vi "Teleop.vi"(10 "Match Info":T3={"Autonomous Elapsed Seconds"=0.0, "TeleOp Elapsed Seconds"=0.0, "Disabled Elapsed Seconds"=0.0, "Visited Autonomous"=FALSE, "Visited TeleOp"=FALSE, "Visited Disabled"=FALSE, "Autonomous Settings"={"Autonomous Style"=enum."Independent", "VI Refnum"=refnum}}, 11 "Call Context":T4) -> ()   [LabVIEW 2017]
doc: "This VI is called for each TeleOp packet received from the DS where the robot is not disabled. It is often used to read from the joysticks and update I/O or to update setpoints for timed control loops. It should complete and return within 20 milliseconds or it may miss DS packets."
uses:
  <vilib>/Rock Robotics/WPI/DriverStation/WPI_DriverStationDerivedRobotMode.ctl
  <vilib>/Rock Robotics/WPI/DriverStation/WPI_DriverStationMatch Info.ctl
  <vilib>/Rock Robotics/WPI/ThirdParty/Phoenix-LabVIEW/Motor Controller/Controls/CTRE_Phoenix_MotorControl_ControlMode.ctl
  <vilib>/Rock Robotics/WPI/Utilities/WPI_GetSetVariantRefNum.vi
  <vilib>/Rock Robotics/WPI/ThirdParty/Phoenix-LabVIEW/Motor Controller/Get/CTRE_Phoenix_MotorController_GetSelectedSensorData.vi
panel:
  in  "newPosition":i32
  out "Velocity":T1(graph)
  out "Position":T2(graph)
  in  "windowSize":i32=1
  in  "Period":u16(ring)=100 items=["Period_1Ms"=1, "Period_2Ms"=2, "Period_5Ms"=5, "Period_10Ms"=10, "Period_20Ms"=20, "Period_25Ms"=25, "Period_50Ms"=50, "Period_100Ms"=100]
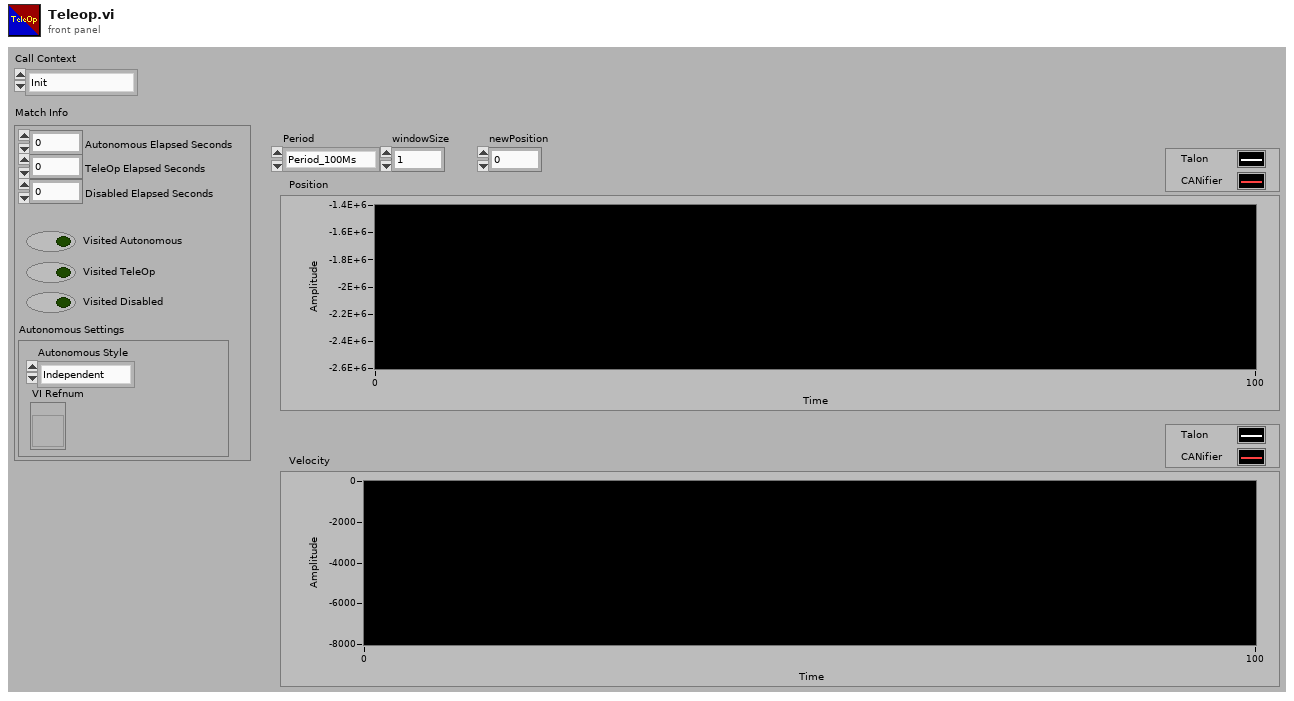
[diagram p1: front panel]
types:
  T1 = cluster{"Velocity (Raw Sensor Units per 100 ms)":i32, "vel":i32}
  T2 = cluster{"Position (Raw Sensor Units)":i32, "pos":i32}
  T3 = typedef "WPI_DriverStationMatch Info.ctl" = cluster{"Autonomous Elapsed Seconds":dbl, "TeleOp Elapsed Seconds":dbl, "Disabled Elapsed Seconds":dbl, "Visited Autonomous":bool, "Visited TeleOp":bool, "Visited Disabled":bool, "Autonomous Settings":cluster{"Autonomous Style":enum16{"Iterative", "Independent"}, "VI Refnum":refnum<vi>}}
  T4 = typedef "WPI_DriverStationDerivedRobotMode.ctl" = enum16{"Init", "Execute", "Stop"}
  T5 = typedef "CTRE_Phoenix_MotorControl_ControlMode.ctl" = u16
  T6 = typedef "WPI_JoystickDevRef.ctl" = cluster{"Device":T7}
  T7 = typedef "WPI_JoystickDeviceEnum.ctl" = enum16{"USB 0", "USB 1", "USB 2", "USB 3", "USB 4", "USB 5"}
  T8 = typedef "CTRE_CANifier_DeviceRef.ctl" = cluster{"DeviceStatus":errorcluster, "Device Number":u8, "Handle":u64, "UsageFrame":u32, "Library Path":path}
  T9 = typedef "WPI_MotorControlDeviceRef.ctl" = cluster{"DeviceStatus":errorcluster, "Type":T10, "PWM":cluster{"PWM Channel":T11, "DeadBand":T12}, "CAN":cluster{"Device Number":u8, "SetOutput VI Ref":variant, "GetOutput VI Ref":variant, "Enable VI Ref":variant, "Disable VI Ref":variant, "Data":variant}, "Invert":bool, "DIO PWM":cluster{"PWM \"Enable\" Channel":T11, "DIOChannel":T13, "PWM Rate":dbl}}
  T10 = typedef "WPI_MotorControlType.ctl" = enum16{"PWM", "CAN", "DIO PWM"}
  T11 = typedef "FPGA_DIOPWMChannel.ctl" = enum8{"PWM 0", "PWM 1", "PWM 2", "PWM 3", "PWM 4", "PWM 5", "PWM 6", "PWM 7", "PWM 8", "PWM 9", "PWM MXP 0", "PWM MXP 1", "PWM MXP 2", "PWM MXP 3", "PWM MXP 4", "PWM MXP 5", "PWM MXP 6", "PWM MXP 7", "PWM MXP 8", "PWM MXP 9", "Invalid"}
  T12 = typedef "WPI_PWMDeadband.ctl" = cluster{"Name":string, "maxPositivePwm":i32, "minPositivePwm":i32, "centerPwm":i32, "maxNegativePwm":i32, "minNegativePwm":i32, "angularRange":u16}
  T13 = typedef "FPGA_DIOChannel.ctl" = enum8{"DIO 0", "DIO 1", "DIO 2", "DIO 3", "DIO 4", "DIO 5", "DIO 6", "DIO 7", "DIO 8", "DIO 9", "DIO MXP 0", "DIO MXP 1", "DIO MXP 2", "DIO MXP 3", "DIO MXP 4", "DIO MXP 5", "DIO MXP 6", "DIO MXP 7", "DIO MXP 8", "DIO MXP 9", "DIO MXP 10", "DIO MXP 11", "DIO MXP 12", "DIO MXP 13", "DIO MXP 14", "DIO MXP 15", "SPI Port CS1", "SPI Port CS2", "SPI Port CS3", "SPI Port MISO", "SPI Port MOSI", "Invalid"}
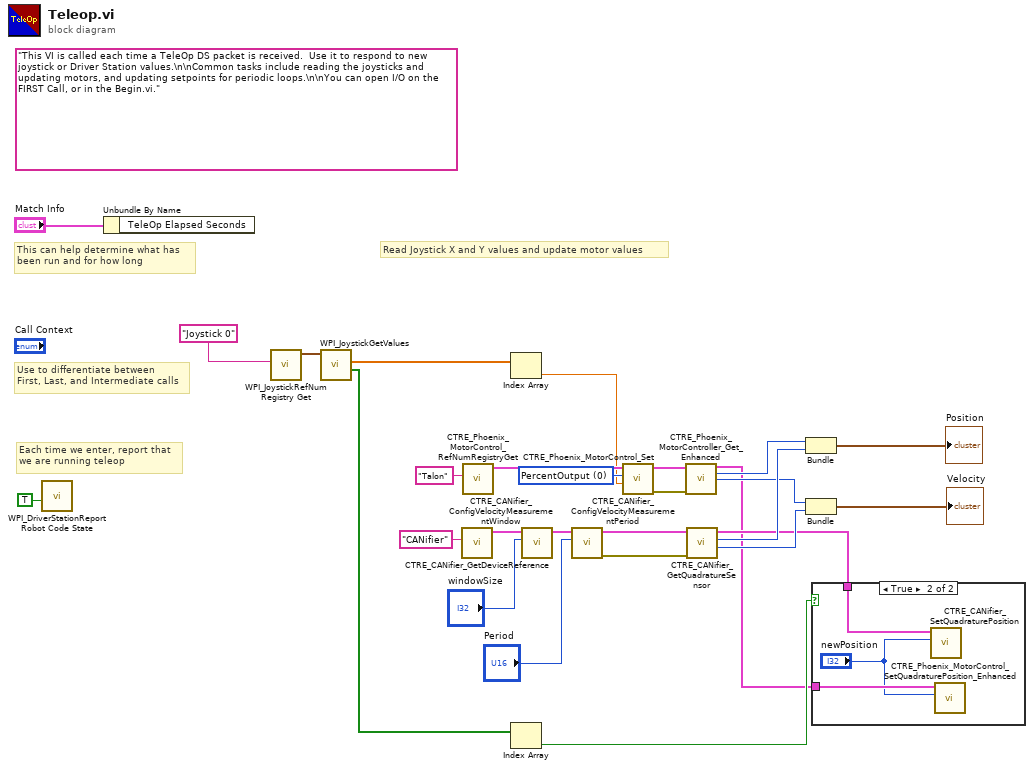
[diagram p0: block diagram]
diagram:
  w20 = T5 0 items=["PercentOutput"=0, "Position"=1, "Velocity"=2, "Current"=3, "Follower"=5, "MotionProfile"=6, "MotionMagic"=7, "MotionMagicArc"=8, "MotionProfileArc"=10, "Disabled"=15] ("Control Mode")
  (unwired) "This VI is called each time a TeleOp DS packet is received.  Use it to respond to new joystick or Driver Station values.\n\nCommon tasks include reading the joysticks and updating motors, and updating setpoints for periodic loops.\n\nYou can open I/O on the FIRST Call, or in the Begin.vi."
  # "Each time we enter, report that\nwe are running teleop"
  # "Use to differentiate between\nFirst, Last, and Intermediate calls"
  # "This can help determine what has\nbeen run and for how long"
  # "Read Joystick X and Y values and update motor values"
  n1 = call <vilib>:"WPI_DriverStationReport Robot Code State.vi"("TeleOp"=TRUE ("Autonomous")) -> ()  [unwired: 10 in, 1 out]
  n2 = Unbundle By Name("Match Info") -> ()  [unwired: 1 out]
  n3 = call <vilib>:"WPI_JoystickRefNum Registry Get.vi"("refnum name"="Joystick 0") -> ("JoystickDevRef"=w26:T6)  [unwired: 1 in, 9 out]
  n4 = call <vilib>:"WPI_JoystickGetValues.vi"("JoystickDevRef"=w26) -> ("Buttons"=w3:bool[], "Axes"=w24:dbl[])  [unwired: 6 in, 3 out]
  n5 = call <vilib>:"CTRE_CANifier_GetDeviceReference.vi"("refnum name"="CANifier") -> ("CANifierDevRef"=w18:T8)  [unwired: 9 in, 1 out]
  n6 = call <vilib>:"CTRE_Phoenix_MotorControl_RefNumRegistryGet.vi"("refnum name"="Talon") -> ("PhoenixMotorControlDevRef"=w21:T9)  [unwired: 9 in, 1 out]
  n7 = Index Array(array=w24) -> (element=w19:dbl)  [unwired: 1 in]
  n8 = Index Array(array=w3) -> (element=w2:bool)  [unwired: 1 in]
  n9 = call <vilib>:"CTRE_CANifier_ConfigVelocityMeasurementWindow.vi"("windowSize"="windowSize", "CANifierDevRef"=w18) -> ("CANifierDevRef"=w15:T8)  [unwired: 8 in, 1 out]
  n10 = call <vilib>:"CTRE_CANifier_ConfigVelocityMeasurementPeriod.vi"("Period"="Period", "CANifierDevRef"=w15) -> ("error out"=w17:errorcluster, "CANifierDevRef"=w16:T8)  [unwired: 8 in]
  n11 = call <vilib>:"CTRE_Phoenix_MotorControl_Set.vi"("Output"=w19, "Control Mode"=w20, "PhoenixMotorControlDevRef"=w21) -> ("error out"=w11:errorcluster, "PhoenixMotorControlDevRef"=w12:T9)  [unwired: 7 in]
  n12 = call-poly <vilib>:"CTRE_Phoenix_MotorController_Get_Enhanced.vi"("PhoenixMotorControlDevRef"=w12, "error in"=w11) -> ("PhoenixMotorControlDevRef"=w1:T9, "Position (Raw Sensor Units)"=w10:i32, "Velocity (Raw Sensor Units per 100 ms)"=w7:i32)  [unwired: 10 in, 1 out]
  n13 = call <vilib>:"CTRE_CANifier_GetQuadratureSensor.vi"("error in"=w17, "CANifierDevRef"=w16) -> ("vel"=w6:i32, "pos"=w9:i32, "CANifierDevRef"=w4:T8)  [unwired: 6 in, 1 out]
  n14 = Bundle("Position (Raw Sensor Units)"=w10, "pos"=w9) -> (→"Position":T2)  [unwired: 1 in]
  n15 = Bundle("Velocity (Raw Sensor Units per 100 ms)"=w7, "vel"=w6) -> (→"Velocity":T1)  [unwired: 1 in]
  n16 = case shown="True" w2 {
    tunnel: w4 -> [_ w31]
    tunnel: w1 -> [_ w30]
    frame False {
    }
    frame True {
      n17 = call <vilib>:"CTRE_CANifier_SetQuadraturePosition.vi"("newPosition"="newPosition", "CANifierDevRef"=w31) -> ()  [unwired: 8 in, 2 out]
      n18 = call <vilib>:"CTRE_Phoenix_MotorControl_SetQuadraturePosition_Enhanced.vi"("New Position"="newPosition", "PhoenixMotorControlDevRef"=w30) -> ()  [unwired: 8 in, 2 out]
    }
  }
